vi "Climb Global.vi"() -> ()   [LabVIEW 2019]
uses:
  Calculations or utilities/Is command done typedef.ctl
  Climb Command Type Def.ctl
  Climb Mode Type Def.ctl
panel:
  out "Climb Mode":T1
  in  "Climb Command":T2
  out "Climb Command Done?":T3
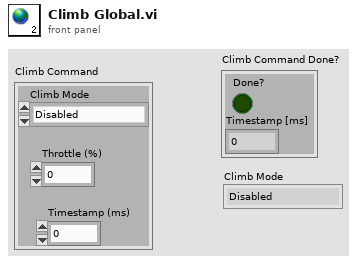
[diagram p1: front panel]
types:
  T1 = typedef "Climb Mode Type Def.ctl" = enum16{"Disabled", "Raw Throttle", "Auto Climb"}
  T2 = typedef "Climb Command Type Def.ctl" = cluster{"Climb Mode":T1, "Throttle (%)":dbl, "Timestamp (ms)":dbl}
  T3 = typedef "Is command done typedef.ctl" = cluster{"Done?":bool, "Timestamp [ms]":dbl}
diagram:
